vi "NJU Project.vi"() -> ()   [LabVIEW 2020]
uses:
  <vilib>/Math Plots/3D Math Plots/3D Surface/3D Surface XCtrl/3D Surface.xctl
  <vilib>/Math Plots/3D Math Plots/3D Surface/3D Surface Datatype/3D Surface Datatype.lvclass
  <vilib>/Math Plots/3D Math Plots/3D Surface/3D Surface Datatype/Public/Plot Helper (Vector).vi
  <vilib>/Utility/inputDevices.llb/closeKeyboard.vi
  lib/Beep/Beep.lvlib
panel:
  out "数据路径":path
  out "Y个数":u16=1 min=1 step=1
  out "X个数":u16=1 min=1 step=1
  out "闪烁分频":u8(slide) scale=0.0..100.0
  out "通道2数据":dbl
  out "通道1数据":dbl
  out "Y索引":i32
  out "X索引":i32
  out "Channel_2_集合":dbl[][](array[numeric])
  out "Channel_1_集合":dbl[][](array[numeric])
  out "Error Info":errorcluster
  out "R偏移":dbl
  in  "数据记录":T1
  out "X偏移":dbl
  out "Y偏移":dbl
  out "R起始":dbl
  out "Y起始":dbl
  out "X起始":dbl
  out "系统状态":bool
  out "R位置":dbl format="%.2f"
  out "Y位置":dbl format="%.6f"
  out "X位置":dbl format="%.6f"
  in  "Main":enum32{"扫描参数设置", "扫描数据预览"}(tab)
  in  "文件名":string="Scan"
  in  "验证":bool
  in  "扫描间距":dbl=2.0 format="%.2f"
  in  "采样率":u16(ring)=11 items=["62.5 mHz", "125 mHz", "250 mHz", "500 mHz", "1 Hz", "2 Hz", "4 Hz", "8Hz", "16 Hz", "32 Hz", "64 Hz", "128 Hz", "256 Hz", "512 Hz", "Trigger "]
  in  "R步进":dbl min=0.0 max=360.0 step=1.0 format="%.2g"
  in  "Y宽度":dbl=10.0 min=0.0 format="%.2f"
  in  "X宽度":dbl=10.0 min=0.0 format="%.2f"
  in  "积分点数":u16=100 min=1 step=1
  in  "R个数":u16=1 min=1 step=1
  in  "R移动":bool
  in  "R角度":dbl min=0.0 max=360.0 step=1.0 format="%.2g"
  in  "SR830":refnum<visa-resource-name>
  out "Logo":picture
  out "通道2预览":refnum<class "3D Plot Datatype.lvclass">[](xcontrol)
  out "通道1":sgl[](graph)
  out "通道2":sgl[](graph)
  out "通道1预览":refnum<class "3D Plot Datatype.lvclass">[](xcontrol)
  in  "扫描":bool
  out "扫描进度(s)":string
  out "扫描进度(%)":u8(slide) scale=0.0..100.0
  out "数据对象":refnum<file>
  out "测量总数":dbl
  out "当前索引":u32(slide) scale=0.0..100.0
  out "开始时间":dbl
  out "键盘设备":refnum<k1> caption="设备ID"
  # "mm"
  # "mm"
  # "偏振光角度"
  # "Step 2 >> 打开激光源并等待至少20分钟\n(衰减片衰减强度调整至最大)\n同时打开白光灯，调整物镜观察样品"
  # "Step 6 >> 衰减片强度调整至合适\n关闭白光灯并注意其他光源干扰\n记录实验数据"
  # "Step 4 >> 寻找样品位置"
  # "上下左右按键\n调整位置"
  # "Step 7 >> 设置数据文件保存名称"
  # "Step 8 >> 开始扫描"
  # "Step 5 >> 设置并验证扫描参数"
  # "XY轴间距一致(μm)"
  # "扫描间距"
  # "采样率"
  # "步进角度(°)"
  # "Y宽度(μm)"
  # "X宽度(μm)"
  # "积分点数"
  # "R扫描个数"
  # "Step 3 >> 调整偏振光角度"
  # "Step 1 >> 选择SR830设备"
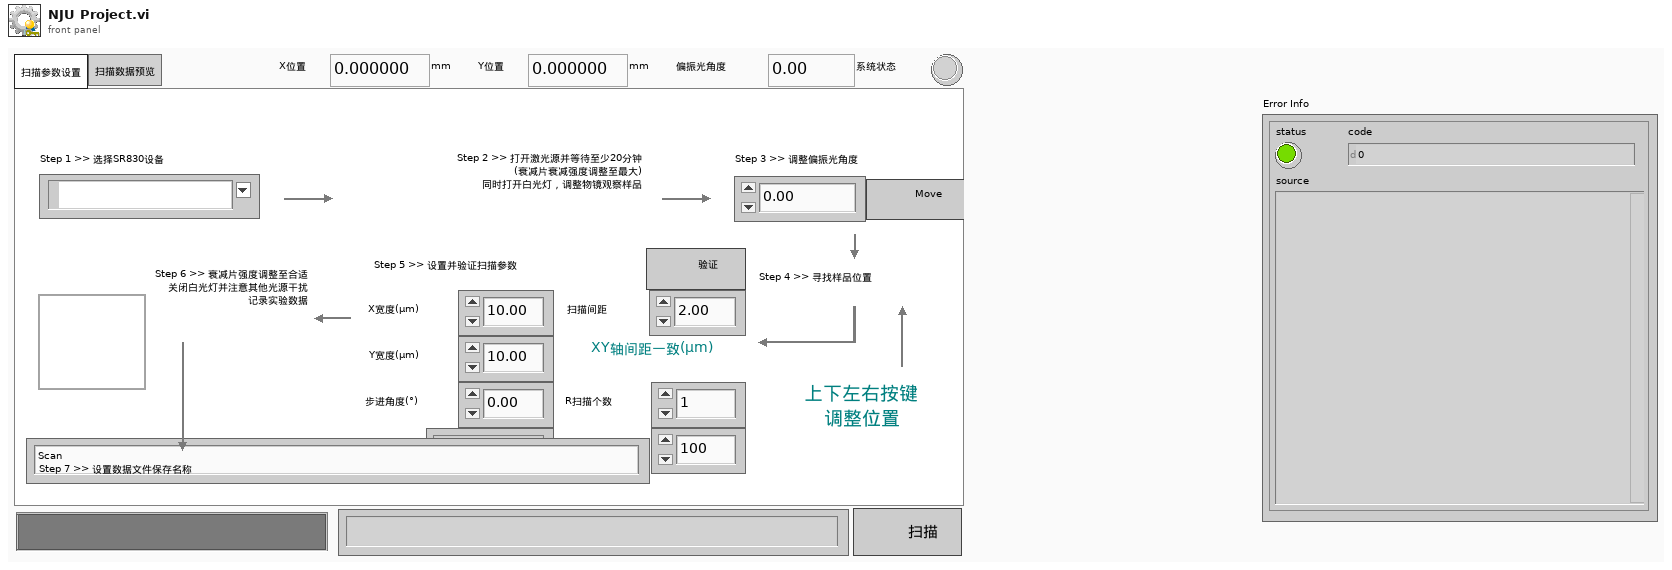
[diagram p1: front panel]
types:
  T1 = cluster{"X轴位置":dbl, "Y轴位置":dbl, "偏振光角度":dbl, "通道1":dbl, "通道2":dbl}
  T2 = typedef "imagedata.ctl" = cluster{"image type":i32, "image depth":i32, "image":u8[], "mask":u8[], "colors":u32[], "Rectangle":cluster{"left":i16, "top":i16, "right":i16, "bottom":i16}}
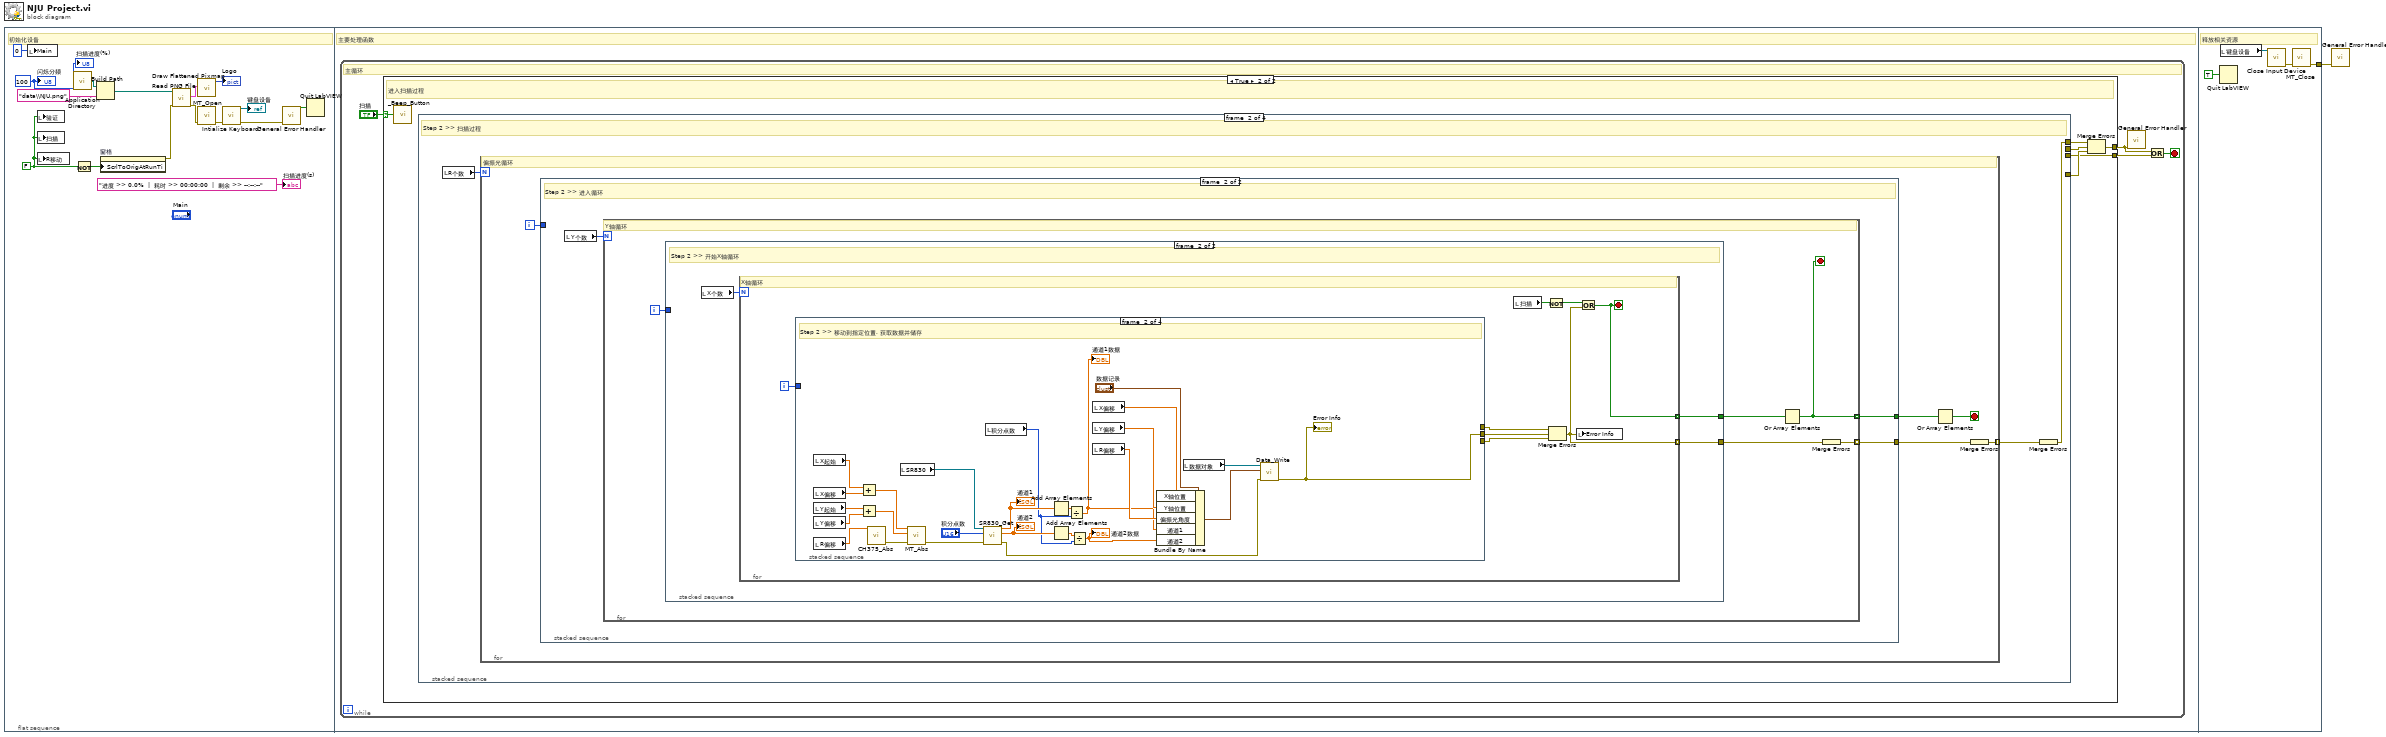
[diagram p0: block diagram]
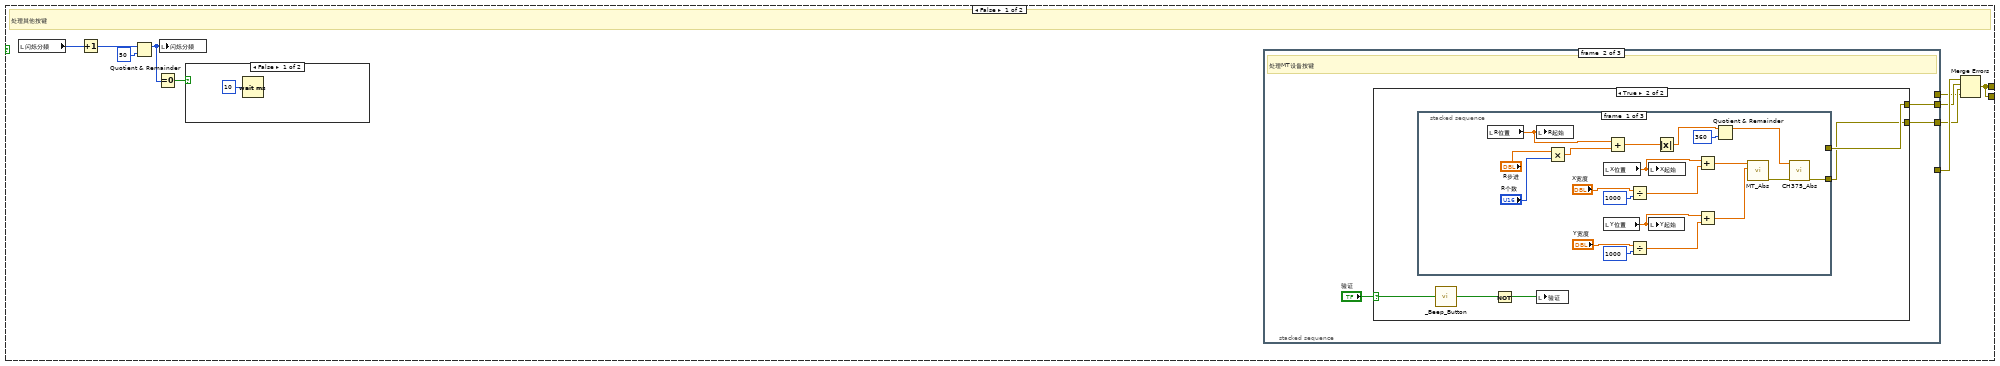
[diagram p2: hidden frame]
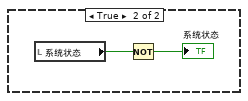
[diagram p3: hidden frame]
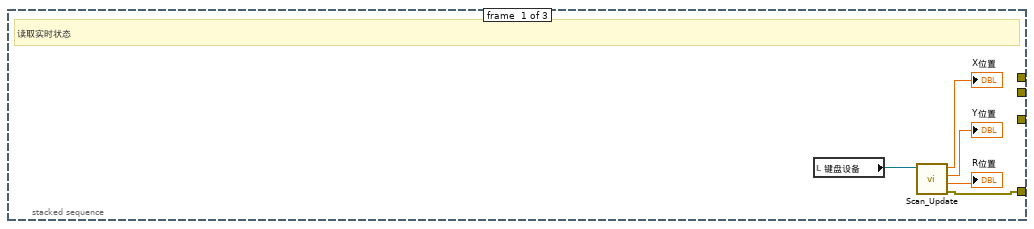
[diagram p4: hidden frame]
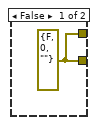
[diagram p5: hidden frame]
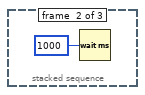
[diagram p6: hidden frame]
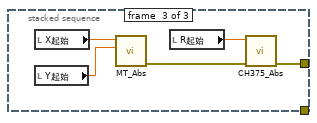
[diagram p7: hidden frame]
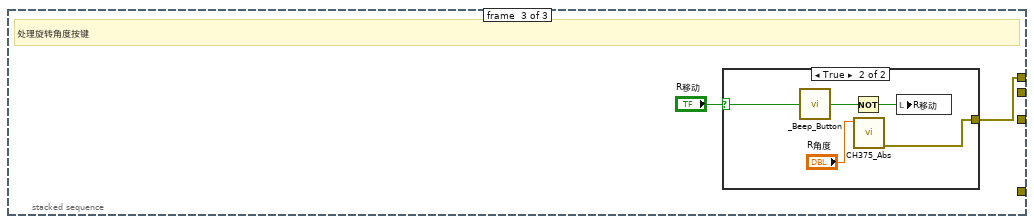
[diagram p8: hidden frame]
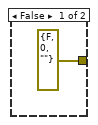
[diagram p9: hidden frame]
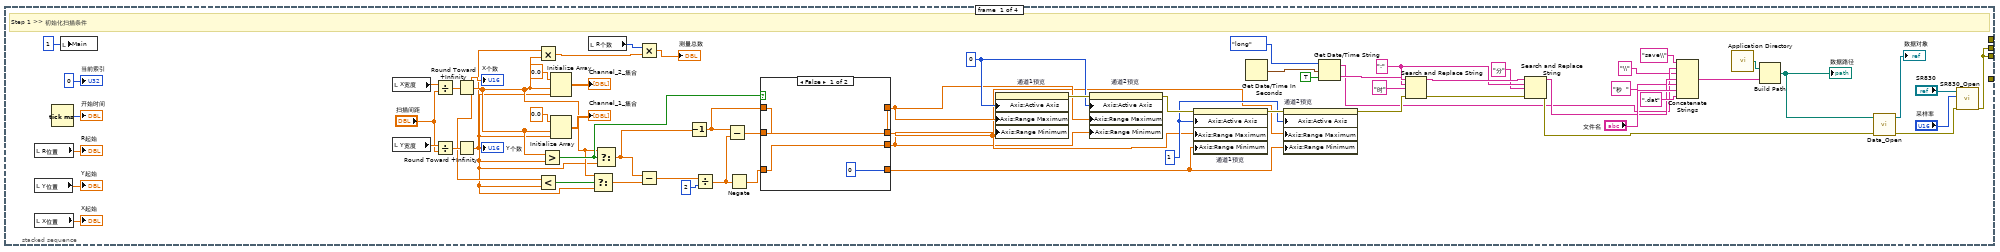
[diagram p10: hidden frame]
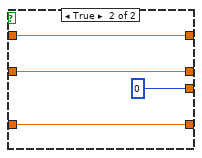
[diagram p11: hidden frame]
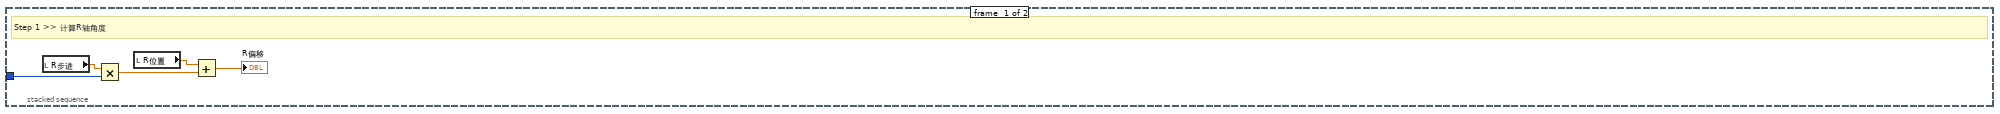
[diagram p12: hidden frame]
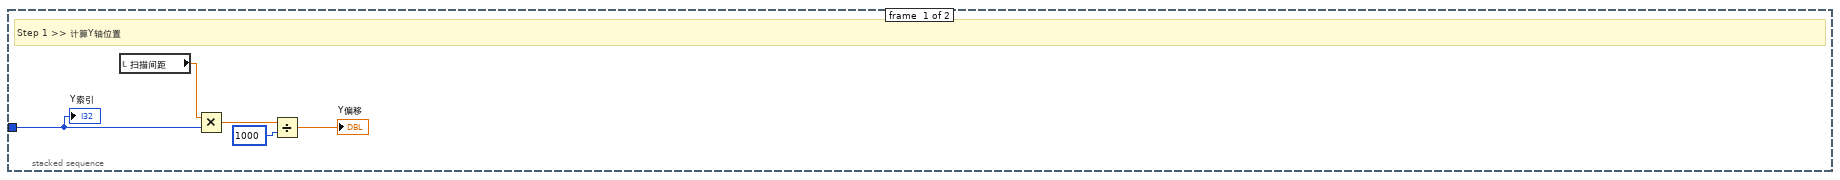
[diagram p13: hidden frame]
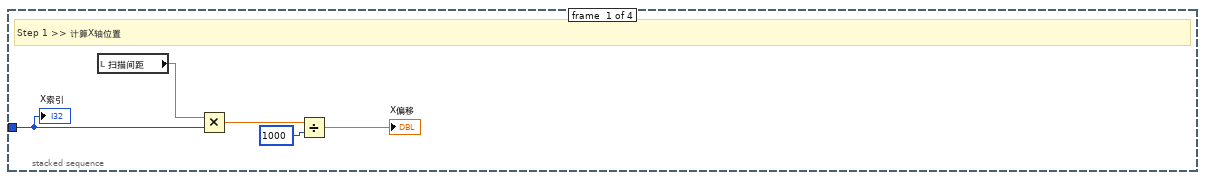
[diagram p14: hidden frame]
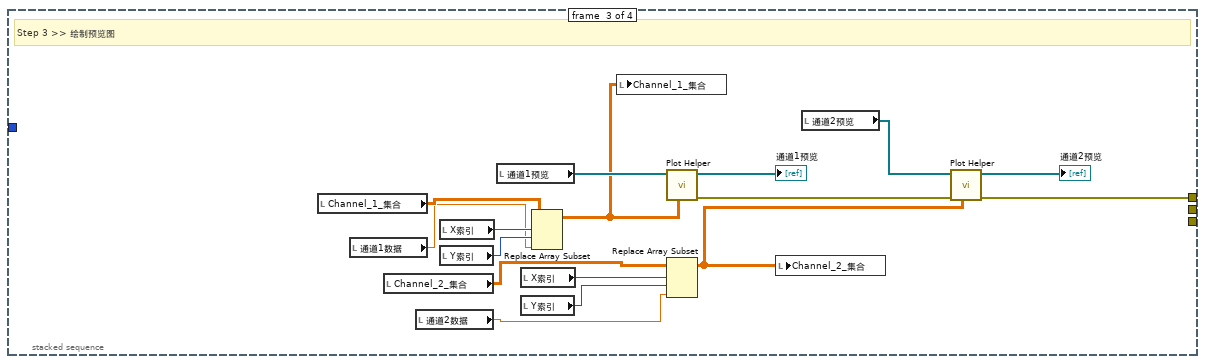
[diagram p15: hidden frame]
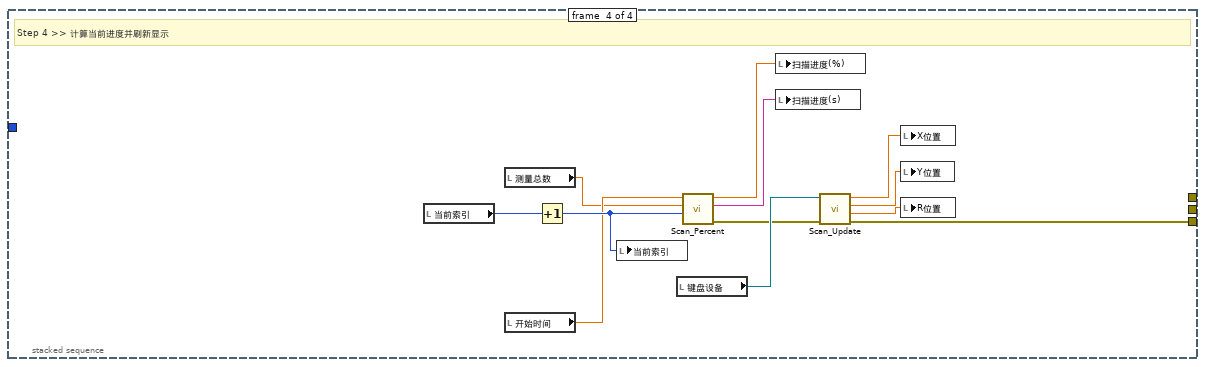
[diagram p16: hidden frame]
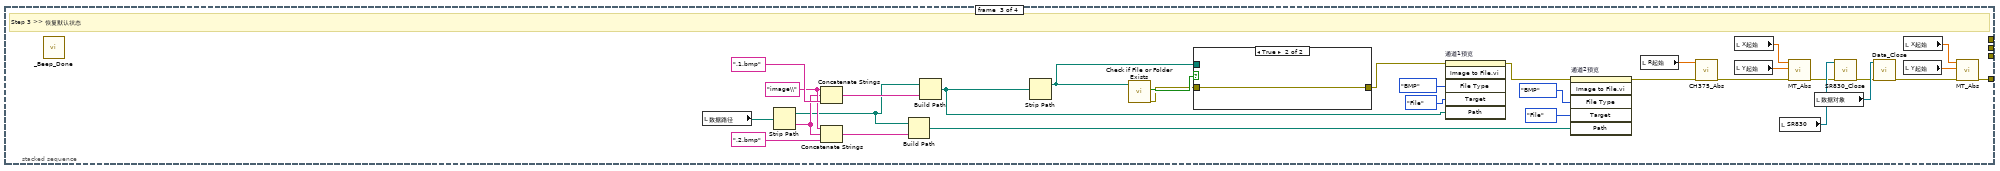
[diagram p17: hidden frame]
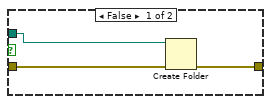
[diagram p18: hidden frame]
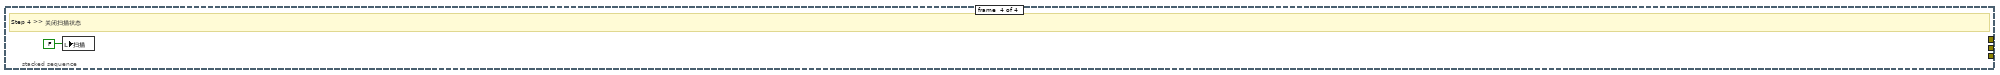
[diagram p19: hidden frame]
diagram:
  n1 = flat-sequence {
    tunnel: [w296] -> w1
    frame #0 {
      w2 = 100
      w4 = FALSE
      # "初始化设备"
      n2 = local write "Main"(0) -> ()
      n3 = local write "验证"(w4) -> ()
      n4 = local write "扫描"(w4) -> ()
      n5 = local write "R移动"(w4) -> ()
      n6 = call <vilib>:"Application Directory.vi"() -> ("Application Directory"=w17:path)
      n7 = Not(x=w4) -> (.not. x?=w8:bool)
      n8 = Build Path(base path=w17, name or relative path="data\\NJU.png") -> (appended path=w13:path)
      n9 = property on="窗格" class="Pane"("ScrlToOrigAtRunTi"=w8) -> (error out=w7:errorcluster)  [unwired: 2 in, 1 out]
      n10 = call <vilib>:"Read PNG File.vi"("error in (no error)"=w7, "path to PNG file"=w13) -> ("error out"=w10:errorcluster, "image data"=w12:T2)  [unwired: 7 in, 1 out]
      n11 = call <vilib>:"Draw Flattened Pixmap.vi"("image data"=w12) -> ("new picture"=→"Logo":picture)  [unwired: 8 in]
      n12 = call "MT_Open.vi"("Error In"=w10) -> ("Error Out"=w15:errorcluster)  [unwired: 9 in, 1 out]
      n13 = call <vilib>:"Intialize Keyboard.vi"("error in (no error)"=w15) -> ("error out"=w9:errorcluster, "device ID"=→"键盘设备":refnum<k1>)  [unwired: 9 in]
      n14 = call <vilib>:"General Error Handler.vi"("error in (no error)"=w9) -> ("error?"=w6:bool)  [unwired: 10 in, 4 out]
      n15 = Quit LabVIEW(quit? (T)=w6) -> ()
      "扫描进度(s)" <- "进度 >> 0.0%  |  耗时 >> 00:00:00  |  剩余 >> --:--:--"
      "扫描进度(%)" <- w2
      "闪烁分频" <- w2
    }
    frame #1 {
      # "主要处理函数"
      n16 = while {
        stop <- w20 stop-if-true
        # "主循环"
        n17 = case shown="True" "扫描" {
          selector: "扫描" -> [_ w88]
          tunnel: [w27 w84] -> w19
          tunnel: [w27 w83] -> w18
          frame False {
            # "处理其他按键"
            n18 = local read "闪烁分频"() -> (w25:u8)
            n19 = Increment(x=w25) -> (x+1=w24:u8)
            n20 = Quotient & Remainder(x=w24, y=50) -> (x-y*floor(x/y)=w23:i32)  [unwired: 1 out]
            n21 = Equal To 0?(x=w23) -> (x = 0?=w22:bool)
            n22 = local write "闪烁分频"(w23) -> ()
            n23 = case shown="False" w22 {
              frame False {
                n24 = Wait (ms)(milliseconds to wait=10) -> ()  [unwired: 1 out]
              }
              frame True {
                n25 = local read "系统状态"() -> (w34:bool)
                n26 = Not(x=w34) -> (.not. x?=→"系统状态":bool)
              }
            }
            n27 = stacked-sequence {
              tunnel: [_ _ w75] -> w28
              tunnel: [w35 _ _] -> w31
              tunnel: [_ w41 _] -> w30
              tunnel: [_ w40 _] -> w29
              frame #0 {
                # "读取实时状态"
                n28 = local read "键盘设备"() -> (w39:refnum<k1>)
                n29 = call "Scan_Update.vi"("键盘设备"=w39) -> ("Error Out"=w35:errorcluster, "偏振光角度"=→"R位置":dbl, "Y轴位置"=→"Y位置":dbl, "X轴位置"=→"X位置":dbl)  [unwired: 7 in]
              }
              frame #1 {
                # "处理MT设备按键"
                n30 = case shown="True" "验证" {
                  selector: "验证" -> [_ w47]
                  tunnel: [w43 w45] -> w41
                  tunnel: [w43 w44] -> w40
                  frame False {
                    w43 = errorcluster {"status"=FALSE, "code"=0, "source"=""} ("error constant")
                  }
                  frame True {
                    n31 = stacked-sequence {
                      tunnel: [_ _ w71] -> w45
                      tunnel: [w50 _ _] -> w44
                      frame #0 {
                        n32 = local read "R位置"() -> (w51:dbl)
                        n33 = local write "R起始"(w51) -> ()
                        n34 = Multiply(x="R步进", y="R个数") -> (x*y=w58:dbl)
                        n35 = local read "X位置"() -> (w54:dbl)
                        n36 = local read "Y位置"() -> (w53:dbl)
                        n37 = Add(x=w51, y=w58) -> (x+y=w57:dbl)
                        n38 = Divide(x="X宽度", y=1000) -> (x/y=w64:dbl)
                        n39 = Divide(x="Y宽度", y=1000) -> (x/y=w62:dbl)
                        n40 = local write "X起始"(w54) -> ()
                        n41 = local write "Y起始"(w53) -> ()
                        n42 = Absolute Value(x=w57) -> (abs(x)=w56:dbl)
                        n43 = Add(x=w54, y=w64) -> (x+y=w67:dbl)
                        n44 = Add(x=w53, y=w62) -> (x+y=w65:dbl)
                        n45 = Quotient & Remainder(x=w56, y=360) -> (x-y*floor(x/y)=w52:dbl)  [unwired: 1 out]
                        n46 = call "MT_Abs.vi"("X轴位置(mm)"=w67, "Y轴位置(mm)"=w65) -> ("Error Out"=w49:errorcluster)  [unwired: 8 in]
                        n47 = call "CH375_Abs.vi"("Error In"=w49, "旋转角度"=w52) -> ("Error Out"=w50:errorcluster)  [unwired: 9 in]
                      }
                      frame #1 {
                        n48 = Wait (ms)(milliseconds to wait=1000) -> ()  [unwired: 1 out]
                      }
                      frame #2 {
                        n49 = local read "X起始"() -> (w72:dbl)
                        n50 = local read "Y起始"() -> (w73:dbl)
                        n51 = call "MT_Abs.vi"("X轴位置(mm)"=w72, "Y轴位置(mm)"=w73) -> ("Error Out"=w70:errorcluster)  [unwired: 8 in]
                        n52 = local read "R起始"() -> (w74:dbl)
                        n53 = call "CH375_Abs.vi"("Error In"=w70, "旋转角度"=w74) -> ("Error Out"=w71:errorcluster)  [unwired: 9 in]
                      }
                    }
                    n54 = call "_Beep_Button.vi"("状态输入"=w47) -> ("状态输出"=w46:bool)  [unwired: 4 in]
                    n55 = Not(x=w46) -> (.not. x?=w48:bool)
                    n56 = local write "验证"(w48) -> ()
                  }
                }
              }
              frame #2 {
                # "处理旋转角度按键"
                n57 = case shown="True" "R移动" {
                  selector: "R移动" -> [_ w81]
                  tunnel: [errorcluster {"status"=FALSE, "code"=0, "source"=""} ("error constant") w79] -> w75
                  frame False {
                  }
                  frame True {
                    n58 = call "_Beep_Button.vi"("状态输入"=w81) -> ("状态输出"=w80:bool)  [unwired: 4 in]
                    n59 = Not(x=w80) -> (.not. x?=w82:bool)
                    n60 = call "CH375_Abs.vi"("旋转角度"="R角度") -> ("Error Out"=w79:errorcluster)  [unwired: 10 in]
                    n61 = local write "R移动"(w82) -> ()
                  }
                }
              }
            }
            n62 = Merge Errors(w31, w30, w29, w28) -> (w27:errorcluster)
          }
          frame True {
            # "进入扫描过程"
            n63 = call "_Beep_Button.vi"("状态输入"=w88) -> ()  [unwired: 4 in, 1 out]
            n64 = stacked-sequence {
              tunnel: [_ w162 _ _] -> w86
              tunnel: [w139 _ _ _] -> w87
              tunnel: [_ _ w283 _] -> w85
              tunnel: [w139 _ _ _] -> w83
              frame #0 {
                w106 = ":"
                w125 = 1
                w126 = 0
                # "Step 1 >> 初始化扫描条件"
                n65 = local read "R位置"() -> (→"R起始":dbl)
                n66 = local read "Y位置"() -> (→"Y起始":dbl)
                n67 = local read "X位置"() -> (→"X起始":dbl)
                n68 = Tick Count (ms)() -> (millisecond timer value=→"开始时间":u32)
                n69 = local write "Main"(1) -> ()
                n70 = local read "X宽度"() -> (w100:dbl)
                n71 = local read "Y宽度"() -> (w99:dbl)
                n72 = Divide(x=w100, y="扫描间距") -> (x/y=w97:dbl)
                n73 = Divide(x=w99, y="扫描间距") -> (x/y=w96:dbl)
                n74 = Round Toward +Infinity(x=w97) -> (ceil(x): smallest int >= x=w95:dbl)
                "X个数" <- w95
                n75 = Round Toward +Infinity(x=w96) -> (ceil(x): smallest int >= x=w94:dbl)
                "Y个数" <- w94
                n76 = Multiply(x=w94, y=w95) -> (x*y=w152:dbl)
                n77 = Less?(x=w95, y=w94) -> (x < y?=w133:bool)
                n78 = Greater?(x=w95, y=w94) -> (0:w124:bool)
                n79 = Initialize Array(0.0, w95, w94) -> (→"Channel_2_集合":dbl[][])
                n80 = Initialize Array(0.0, w95, w94) -> (→"Channel_1_集合":dbl[][])
                n81 = local read "R个数"() -> (w151:u16)
                n82 = Select(t=w95, s=w133, f=w94) -> (s? t:f=w132:dbl)
                n83 = Select(t=w95, s=w124, f=w94) -> (s? t:f=w116:dbl)
                n84 = Multiply(x=w151, y=w152) -> (x*y=→"测量总数":dbl)
                n85 = Subtract(x=w116, y=w132) -> (x-y=w131:dbl)
                n86 = Decrement(x=w116) -> (x-1=w89:dbl)
                n87 = Divide(x=w131, y=2) -> (x/y=w119:dbl)
                n88 = Subtract(x=w89, y=w119) -> (x-y=w122:dbl)
                n89 = Negate(x=w119) -> (-x=w118:dbl)
                n90 = case shown="False" w124 {
                  tunnel: w89 -> [w155 w161]
                  tunnel: [w157 w161] -> w123
                  tunnel: w122 -> [w157 w160]
                  tunnel: [w155 w160] -> w121
                  tunnel: [w156 0] -> w120
                  tunnel: [0 w158] -> w117
                  tunnel: w118 -> [w156 w158]
                  frame False {
                  }
                  frame True {
                  }
                }
                n91 = property on="通道1预览" class="3D Surface (strict)"("Axis:Active Axis"=w126, "Axis:Range Maximum"=w123, "Axis:Range Minimum"=w120) -> (error out=w128:errorcluster)  [unwired: 2 in, 1 out]
                n92 = property on="通道2预览" class="3D Surface (strict)"(error in=w128, "Axis:Active Axis"=w126, "Axis:Range Maximum"=w123, "Axis:Range Minimum"=w120) -> (error out=w127:errorcluster)  [unwired: 1 in, 1 out]
                n93 = property on="通道1预览" class="3D Surface (strict)"(error in=w127, "Axis:Active Axis"=w125, "Axis:Range Maximum"=w121, "Axis:Range Minimum"=w117) -> (error out=w129:errorcluster)  [unwired: 1 in, 1 out]
                n94 = Get Date/Time In Seconds() -> (seconds since 1Jan1904=w115:timestamp)
                n95 = property on="通道2预览" class="3D Surface (strict)"(error in=w129, "Axis:Active Axis"=w125, "Axis:Range Maximum"=w121, "Axis:Range Minimum"=w117) -> (error out=w108:errorcluster)  [unwired: 1 in, 1 out]
                n96 = Get Date/Time String(date format (0)=enum16{"short", "long", "abbreviated"}."long", seconds (now)=w115, want seconds? (F)=TRUE) -> (date string=w91:string, time string=w112:string)
                n97 = Search and Replace String(input string=w112, search string=w106, replace string="时", error in=w108) -> (result string=w107:string, error out=w104:errorcluster)  [unwired: 4 in, 2 out]
                n98 = Search and Replace String(input string=w107, search string=w106, replace string="分", error in=w104) -> (result string=w102:string, error out=w103:errorcluster)  [unwired: 4 in, 2 out]
                n99 = Concatenate Strings("save\\", w91, "\\", w102, "秒  ", "文件名", ".dat") -> (w147:string)
                n100 = call <vilib>:"Application Directory.vi"() -> ("Application Directory"=w146:path)
                n101 = Build Path(base path=w146, name or relative path=w147) -> (appended path=w93:path)
                "数据路径" <- w93
                n102 = call "Data_Open.vi"("Error In"=w103, "文件路径（使用对话框）"=w93) -> ("Error Out"=w140:errorcluster, "数据文件对象"=→"数据对象":refnum<file>)  [unwired: 8 in]
                n103 = call "SR830_Open.vi"("Error In"=w140, "Sample Rate (0: 62.5 mHz)"="采样率", "VISA 输入"="SR830") -> ("Error Out"=w139:errorcluster)  [unwired: 8 in]
                "当前索引" <- 0
              }
              frame #1 {
                # "Step 2 >> 扫描过程"
                n104 = local read "R个数"() -> (w163:u16)
                n105 = for {
                  N: w163 -> [_]
                  tunnel: [w168] -> w164 mode=indexing
                  i -> [w165]
                  stop <- w166 stop-if-true
                  # "偏振光循环"
                  n106 = stacked-sequence {
                    tunnel: w165 -> [w170 _]
                    tunnel: [_ w177] -> w169
                    tunnel: [_ w175] -> w167
                    frame #0 {
                      # "Step 1 >> 计算R轴角度"
                      n107 = local read "R步进"() -> (w174:dbl)
                      n108 = Multiply(x=w174, y=w170) -> (x*y=w172:dbl)
                      n109 = local read "R位置"() -> (w173:dbl)
                      n110 = Add(x=w173, y=w172) -> (x+y=→"R偏移":dbl)
                    }
                    frame #1 {
                      # "Step 2 >> 进入循环"
                      n111 = local read "Y个数"() -> (w176:u16)
                      n112 = for {
                        N: w176 -> [_]
                        tunnel: [w182] -> w177 mode=indexing
                        tunnel: [w181] -> w175 mode=indexing
                        i -> [w178]
                        stop <- w181 stop-if-true
                        # "Y轴循环"
                        n113 = stacked-sequence {
                          tunnel: w178 -> [w183 _]
                          tunnel: [_ w190] -> w180
                          tunnel: [_ w188] -> w179
                          frame #0 {
                            # "Step 1 >> 计算Y轴位置"
                            n114 = local read "扫描间距"() -> (w184:dbl)
                            n115 = Multiply(x=w184, y=w183) -> (x*y=w185:dbl)
                            n116 = Divide(x=w185, y=1000) -> (x/y=→"Y偏移":dbl)
                            "Y索引" <- w183
                          }
                          frame #1 {
                            # "Step 2 >> 开始X轴循环"
                            n117 = local read "X个数"() -> (w189:u16)
                            n118 = for {
                              N: w189 -> [_]
                              tunnel: [w195] -> w190 mode=indexing
                              tunnel: [w192] -> w188 mode=indexing
                              i -> [w198]
                              stop <- w195 stop-if-true
                              # "X轴循环"
                              n119 = stacked-sequence {
                                tunnel: w198 -> [w199 _ _ _]
                                tunnel: [_ w220 _ _] -> w194
                                tunnel: [_ _ _ w246] -> w193
                                tunnel: [_ _ w241 _] -> w191
                                frame #0 {
                                # "Step 1 >> 计算X轴位置"
                                n120 = local read "扫描间距"() -> (w202:dbl)
                                n121 = Multiply(x=w202, y=w199) -> (x*y=w203:dbl)
                                n122 = Divide(x=w203, y=1000) -> (x/y=→"X偏移":dbl)
                                "X索引" <- w199
                                }
                                frame #1 {
                                # "Step 2 >> 移动到指定位置, 获取数据并储存"
                                n123 = local read "X起始"() -> (w217:dbl)
                                n124 = local read "X偏移"() -> (w211:dbl)
                                n125 = local read "Y起始"() -> (w216:dbl)
                                n126 = local read "Y偏移"() -> (w213:dbl)
                                n127 = local read "R偏移"() -> (w212:dbl)
                                n128 = Add(x=w217, y=w211) -> (x+y=w214:dbl)
                                n129 = Add(x=w216, y=w213) -> (x+y=w215:dbl)
                                n130 = call "CH375_Abs.vi"("旋转角度"=w212) -> ("Error Out"=w218:errorcluster)  [unwired: 10 in]
                                n131 = local read "SR830"() -> (w229:refnum<visa-resource-name>)
                                n132 = call "MT_Abs.vi"("X轴位置(mm)"=w214, "Y轴位置(mm)"=w215, "Error In"=w218) -> ("Error Out"=w210:errorcluster)  [unwired: 7 in]
                                n133 = call "SR830_Get.vi"("Error In"=w210, "数据长度"="积分点数", "VISA 输入"=w229) -> ("Error Out"=w209:errorcluster, "Channel 2"=w227:sgl[], "Channel 1"=w226:sgl[])  [unwired: 6 in]
                                "通道1" <- w226
                                "通道2" <- w227
                                n134 = local read "积分点数"() -> (w204:u16)
                                n135 = Add Array Elements(numeric array=w226) -> (sum=w208:sgl)
                                n136 = Add Array Elements(numeric array=w227) -> (sum=w206:sgl)
                                n137 = Divide(x=w208, y=w204) -> (x/y=w207:sgl)
                                "通道1数据" <- w207
                                n138 = Divide(x=w206, y=w204) -> (x/y=w205:sgl)
                                "通道2数据" <- w205
                                n139 = local read "X偏移"() -> (w223:dbl)
                                n140 = local read "Y偏移"() -> (w222:dbl)
                                n141 = local read "R偏移"() -> (w221:dbl)
                                n142 = Bundle By Name(cluster="数据记录", "X轴位置"=w223, "Y轴位置"=w222, "偏振光角度"=w221, "通道1"=w207, "通道2"=w205) -> (w224:T1)
                                n143 = local read "数据对象"() -> (w228:refnum<file>)
                                n144 = call "Data_Write.vi"("Error In"=w209, "扫描参数"=w224, "数据文件对象"=w228) -> ("Error Out"=w220:errorcluster)  [unwired: 8 in]
                                "Error Info" <- w220
                                }
                                frame #2 {
                                # "Step 3 >> 绘制预览图"
                                n145 = local read "Channel_1_集合"() -> (w239:dbl[][])
                                n146 = local read "通道1数据"() -> (w236:dbl)
                                n147 = local read "Channel_2_集合"() -> (w232:dbl[][])
                                n148 = local read "通道2数据"() -> (w235:dbl)
                                n149 = local read "X索引"() -> (w238:i32)
                                n150 = local read "Y索引"() -> (w237:i32)
                                n151 = local read "通道1预览"() -> (w245:refnum<class "3D Plot Datatype.lvclass">[])
                                n152 = local read "X索引"() -> (w233:i32)
                                n153 = local read "Y索引"() -> (w234:i32)
                                n154 = Replace Array Subset(array=w239, new element=w236, index (row)=w238, index (col)=w237) -> (w231:dbl[][])
                                n155 = local write "Channel_1_集合"(w231) -> ()
                                n156 = call-poly <vilib>:"Plot Helper.vi"("z matrix"=w231, "3D Plot lvclass Array in"=w245) -> ("error out"=w242:errorcluster, "3D Plot lvclass Array out"=→"通道1预览":refnum<class "3D Plot Datatype.lvclass">[])  [unwired: 4 in, 4 out]
                                n157 = Replace Array Subset(array=w232, new element=w235, index (row)=w233, index (col)=w234) -> (w230:dbl[][])
                                n158 = local write "Channel_2_集合"(w230) -> ()
                                n159 = local read "通道2预览"() -> (w243:refnum<class "3D Plot Datatype.lvclass">[])
                                n160 = call-poly <vilib>:"Plot Helper.vi"("z matrix"=w230, "error in (no error)"=w242, "3D Plot lvclass Array in"=w243) -> ("error out"=w241:errorcluster, "3D Plot lvclass Array out"=→"通道2预览":refnum<class "3D Plot Datatype.lvclass">[])  [unwired: 3 in, 4 out]
                                }
                                frame #3 {
                                # "Step 4 >> 计算当前进度并刷新显示"
                                n161 = local read "当前索引"() -> (w257:u32)
                                n162 = local read "测量总数"() -> (w252:dbl)
                                n163 = local read "开始时间"() -> (w255:dbl)
                                n164 = Increment(x=w257) -> (x+1=w256:u32)
                                n165 = local write "当前索引"(w256) -> ()
                                n166 = local read "键盘设备"() -> (w251:refnum<k1>)
                                n167 = call "Scan_Percent.vi"("开始时间"=w255, "测量总数"=w252, "当前索引"=w256) -> ("当前进度(%)"=w254:dbl, "当前进度"=w253:string, "Error Out"=w247:errorcluster)  [unwired: 5 in]
                                n168 = local write "扫描进度(%)"(w254) -> ()
                                n169 = local write "扫描进度(s)"(w253) -> ()
                                n170 = call "Scan_Update.vi"("Error In"=w247, "键盘设备"=w251) -> ("Error Out"=w246:errorcluster, "偏振光角度"=w248:dbl, "Y轴位置"=w249:dbl, "X轴位置"=w250:dbl)  [unwired: 6 in]
                                n171 = local write "X位置"(w250) -> ()
                                n172 = local write "Y位置"(w249) -> ()
                                n173 = local write "R位置"(w248) -> ()
                                }
                              }
                              n174 = local read "扫描"() -> (w197:bool)
                              n175 = Not(x=w197) -> (.not. x?=w196:bool)
                              n176 = Merge Errors(w191, w194, w193) -> (w192:errorcluster)
                              n177 = local write "Error Info"(w192) -> ()
                              n178 = Or(x=w196, y=w192) -> (x .or. y?=w195:bool)
                            }
                          }
                        }
                        n179 = Or Array Elements(Boolean array=w180) -> (logical OR=w181:bool)
                        n180 = Merge Errors(w179) -> (w182:errorcluster)
                      }
                    }
                  }
                  n181 = Or Array Elements(Boolean array=w167) -> (logical OR=w166:bool)
                  n182 = Merge Errors(w169) -> (w168:errorcluster)
                }
                n183 = Merge Errors(w164) -> (w162:errorcluster)
              }
              frame #2 {
                w263 = "image\\"
                # "Step 3 >> 恢复默认状态"
                n184 = call "_Beep_Done.vi"() -> ()  [unwired: 5 in, 1 out]
                n185 = local read "数据路径"() -> (w275:path)
                n186 = Strip Path(path=w275) -> (stripped path=w259:path, name=w262:string)
                n187 = Concatenate Strings(w263, w262, ".1.bmp") -> (w274:string)
                n188 = Concatenate Strings(w263, w262, ".2.bmp") -> (w260:string)
                n189 = Build Path(base path=w259, name or relative path=w260) -> (appended path=w258:path)
                n190 = Build Path(base path=w259, name or relative path=w274) -> (appended path=w269:path)
                n191 = Strip Path(path=w269) -> (stripped path=w267:path)  [unwired: 1 out]
                n192 = call <vilib>:"Check if File or Folder Exists.vi"("path"=w267) -> ("error out"=w265:errorcluster, "file or folder exists?"=w268:bool)  [unwired: 8 in, 1 out]
                n193 = case shown="True" w268 {
                  tunnel: w267 -> [w292 _]
                  tunnel: [w291 w293] -> w266
                  tunnel: w265 -> [w290 w293]
                  frame False {
                    n194 = Create Folder(path (use dialog)=w292, error in=w290) -> (error out=w291:errorcluster)  [unwired: 1 in, 2 out]
                  }
                  frame True {
                  }
                }
                n195 = invoke on="通道1预览" class="3D Surface (strict)" method="Image to File.vi"(error in=w266, "File Type"=enum32{"BMP", "EPS", "EMF", "PICT"}."BMP", "Target"=enum32{"File", "Clipboard"}."File", "Path"=w269) -> (error out=w264:errorcluster)  [unwired: 2 in, 5 out]
                n196 = invoke on="通道2预览" class="3D Surface (strict)" method="Image to File.vi"(error in=w264, "File Type"=enum32{"BMP", "EPS", "EMF", "PICT"}."BMP", "Target"=enum32{"File", "Clipboard"}."File", "Path"=w258) -> (error out=w271:errorcluster)  [unwired: 2 in, 5 out]
                n197 = local read "R起始"() -> (w282:dbl)
                n198 = call "CH375_Abs.vi"("Error In"=w271, "旋转角度"=w282) -> ("Error Out"=w279:errorcluster)  [unwired: 9 in]
                n199 = local read "X起始"() -> (w281:dbl)
                n200 = local read "Y起始"() -> (w280:dbl)
                n201 = local read "SR830"() -> (w285:refnum<visa-resource-name>)
                n202 = call "MT_Abs.vi"("X轴位置(mm)"=w281, "Y轴位置(mm)"=w280, "Error In"=w279) -> ("Error Out"=w278:errorcluster)  [unwired: 7 in]
                n203 = local read "数据对象"() -> (w287:refnum<file>)
                n204 = call "SR830_Close.vi"("Error In"=w278, "VISA 输入"=w285) -> ("Error Out"=w284:errorcluster)  [unwired: 9 in]
                n205 = call "Data_Close.vi"("Error In"=w284, "数据对象保存"=w287) -> ("Error Out"=w286:errorcluster)  [unwired: 9 in]
                n206 = local read "X起始"() -> (w289:dbl)
                n207 = local read "Y起始"() -> (w288:dbl)
                n208 = call "MT_Abs.vi"("X轴位置(mm)"=w289, "Y轴位置(mm)"=w288, "Error In"=w286) -> ("Error Out"=w283:errorcluster)  [unwired: 7 in]
              }
              frame #3 {
                # "Step 4 >> 关闭扫描状态"
                n209 = local write "扫描"(FALSE) -> ()
              }
            }
            n210 = Merge Errors(w86, w87, w85) -> (w84:errorcluster)
          }
        }
        n211 = call <vilib>:"General Error Handler.vi"("error in (no error)"=w19) -> ()  [unwired: 10 in, 5 out]
        n212 = Or(x=w19, y=w18) -> (x .or. y?=w20:bool)
      }
    }
    frame #2 {
      # "释放相关资源"
      n213 = Quit LabVIEW(quit? (T)=TRUE) -> ()
      n214 = local read "键盘设备"() -> (w298:refnum<k1>)
      n215 = call-poly <vilib>:"Close Input Device.vi"("device ID"=w298) -> ("error out"=w297:errorcluster)  [unwired: 9 in]
      n216 = call "MT_Close.vi"("Error In"=w297) -> ("Error Out"=w296:errorcluster)  [unwired: 10 in]
    }
  }
  n217 = call <vilib>:"General Error Handler.vi"("error in (no error)"=w1) -> ()  [unwired: 10 in, 5 out]
